vi "tcpwritearray.vi"(7 "command cluster":T2={"command"=enum."Idle", "start time (ms)"=0, "Channel Indices"=[], "Scans per Sample"=1} {"Scans per Sample" min=1}, 8 "buffer size":i32, 9 "timeout ms (25000)":i32=25000, 10 "data":T4={"voltage data"=[0.0, 0.0, 0.0, 0.0, 0.0, 0.0048828125, 0.0, 0.0, 0.0, 0.0, 0.0024414062, 0.0024414062, 0.0, 0.0, 0.0, 0.0024414062, 0.0, 0.0048828125, 0.0024414062, 0.0048828125, 0.0, 0.0024414062, 0.0024414062, 0.0048828125, 0.01953125, 0.017089844, 0.012207031, 0.0146484375, 0.0146484375, 0.0146484375, 0.01953125, 0.009765625], "seconds since 1904"=0.0, "arbtrary scans"=0} {"seconds since 1904" format="%<%I:%M:%S %p\n%m/%d/%Y>T"; "voltage data" format="%.4f"}, 11 "refnum in":refnum<k5>) -> (0 "error out":errorcluster, 2 "bytes written":i32, 3 "refnum out":refnum<k5>)   [LabVIEW 2012]
uses:
  DataServer/data w time.ctl
  DataServer/command cluster.ctl
  DataServer/command.ctl
  DataServer/data send.ctl
panel:
  in  "all channels":T1={"voltage data"=[0.0, 0.0, 0.0, 0.0, 0.0, 0.0048828125, 0.0, 0.0, 0.0, 0.0, 0.0024414062, 0.0024414062, 0.0, 0.0, 0.0, 0.0024414062, 0.0, 0.0048828125, 0.0024414062, 0.0048828125, 0.0, 0.0024414062, 0.0024414062, 0.0048828125, 0.01953125, 0.017089844, 0.012207031, 0.0146484375, 0.0146484375, 0.0146484375, 0.01953125, 0.009765625], "scan backlog"=0, "seconds since 1904"=0.0, "arbitrary scans"=0} {"seconds since 1904" format="%.2f"; "voltage data" format="%.4f"}
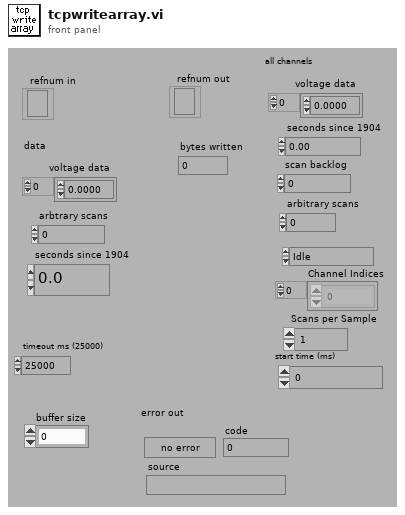
[diagram p1: front panel]
types:
  T1 = typedef "data send.ctl" = cluster{"voltage data":sgl[], "scan backlog":u32, "seconds since 1904":dbl, "arbitrary scans":i32}
  T2 = typedef "command cluster.ctl" = cluster{"command":T3, "start time (ms)":u32, "Channel Indices":i32[], "Scans per Sample":i32}
  T3 = typedef "command.ctl" = enum16{"Idle", "Send Data", "Send 1 Scan", "Logoff"}
  T4 = typedef "data w time.ctl" = cluster{"voltage data":sgl[], "seconds since 1904":dbl, "arbtrary scans":u32}
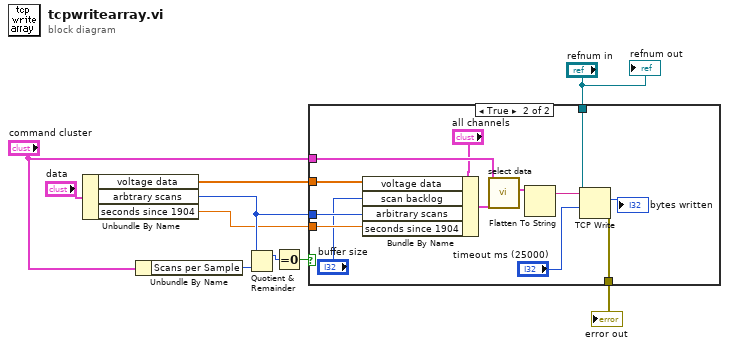
[diagram p0: block diagram]
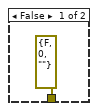
[diagram p2: hidden frame]
diagram:
  n1 = Unbundle By Name("data") -> ("voltage data"=w9:sgl[], "arbtrary scans"=w3:u32, "seconds since 1904"=w2:dbl)
  n2 = Unbundle By Name("command cluster") -> ("Scans per Sample"=w6:i32)
  n3 = Quotient & Remainder(x=w3, y=w6) -> (x-y*floor(x/y)=w7:u32)  [unwired: 1 out]
  n4 = Equal To 0?(x=w7) -> (x = 0?=w8:bool)
  n5 = case shown="True" w8 {
    tunnel: [errorcluster {"status"=FALSE, "code"=0, "source"=""} ("error out") w22] -> w5
    tunnel: "command cluster" -> [_ w20]
    tunnel: w9 -> [_ w16]
    tunnel: w3 -> [_ w15]
    tunnel: w2 -> [_ w14]
    tunnel: "refnum in" -> [_ w13]
    frame False {
    }
    frame True {
      n6 = Bundle By Name(cluster="all channels", "voltage data"=w16, "scan backlog"="buffer size", "arbitrary scans"=w15, "seconds since 1904"=w14) -> (w18:T1)
      n7 = call "select data.vi"("all channels"=w18, "command cluster"=w20) -> ("selected channels"=w19:T1)  [unwired: 9 in]
      n8 = Flatten To String(anything=w19) -> (data string=w21:string)  [unwired: 3 in, 2 out]
      n9 = TCP Write(connection ID=w13, data in=w21, 9:"timeout ms (25000)") -> (bytes written=→"bytes written":i32, error out=w22:errorcluster)  [unwired: 1 in, 1 out]
    }
  }
  "error out" <- w5
  "refnum out" <- "refnum in"
